vi "QPlus_Analyzer 2.0.vi"() -> ()   [LabVIEW 2016]
uses:
  <instrlib>/Stanford Research 830/Public/Data/Read (1 Parameter).vi
  <vilib>/express/express shared/transition.llb/Dynamic To Waveform Array.vi
  <vilib>/express/express signal manip/GetorSetDDTAttributes/Set DDT Attributes/SetT0.vi
  <vilib>/express/express shared/transition.llb/Waveform Array To Dynamic.vi
  <vilib>/express/express signal manip/GetorSetDDTAttributes/Set DDT Attributes/Set DDT Properties.xnode
  <instrlib>/Stanford Research 830/Stanford Research 830.lvlib
  <instrlib>/Agilent 3352X Series/Agilent 3352X Series.lvlib
panel:
  out "Y Signal":cluster{"Y":dbl[], "Y":dbl[]}[](graph)
  out "X Signal":cluster{"Y":dbl[], "Y":dbl[]}[](graph)
  in  "Reference name":refnum<visa-resource-name>
  in  "VISA resource name":refnum<visa-resource-name>
  in  "Sensitivity (26: 1 V/uA)":i8(ring)=26 items=["Auto Gain"=-1, "2 nV/fA"=0, "5 nV/fA"=1, "10 nV/fA"=2, "20 nV/fA"=3, "50 nV/fA"=4, "100 nV/fA"=5, "200 nV/fA"=6, "500 nV/fA"=7, "1 uV/pA"=8, "2 uV/pA"=9, "5 uV/pA"=10, "10 uV/pA"=11, "20 uV/pA"=12, "50 uV/pA"=13, "100 uV/pA"=14, "200 uV/pA"=15, "500 uV/pA"=16, "1 mV/nA"=17, "2 mV/nA"=18, "5 mV/nA"=19, "10 mV/nA"=20, "20 mV/nA"=21, "50 mV/nA"=22, "100 mV/nA"=23, "200 mV/nA"=24, "500 mV/mA"=25, "1 V/uA"=26]
  in  "Time Constant (8: 100ms)":u16(ring)=8 items=["10 us", "30 us", "100 us", "300 us", "1 ms", "3 ms", "10 ms", "30 ms", "100 ms", "300 ms", "1 s", "3 s", "10 s", "30 s", "100 s", "300 s", "1 ks", "3 ks", "10 ks", "30 ks"]
  in  "Save File Name":path=path "G:/UCB/Instruments/tip making/Qplus AFM tip making/qplus test/Caihong/CJ39.xlsx" caption="Filename"
  in  "Time Between Points (sec)":dbl=0.05 format="%#_1f"
  in  "Sine Output Amplitude (1 V)":dbl=1.0
  in  "Starting Frequency (Hz)":dbl=32000.0
  in  "Final Frequency (Hz)":dbl=33000.0
  in  "Step Size (Hz)":dbl=10.0
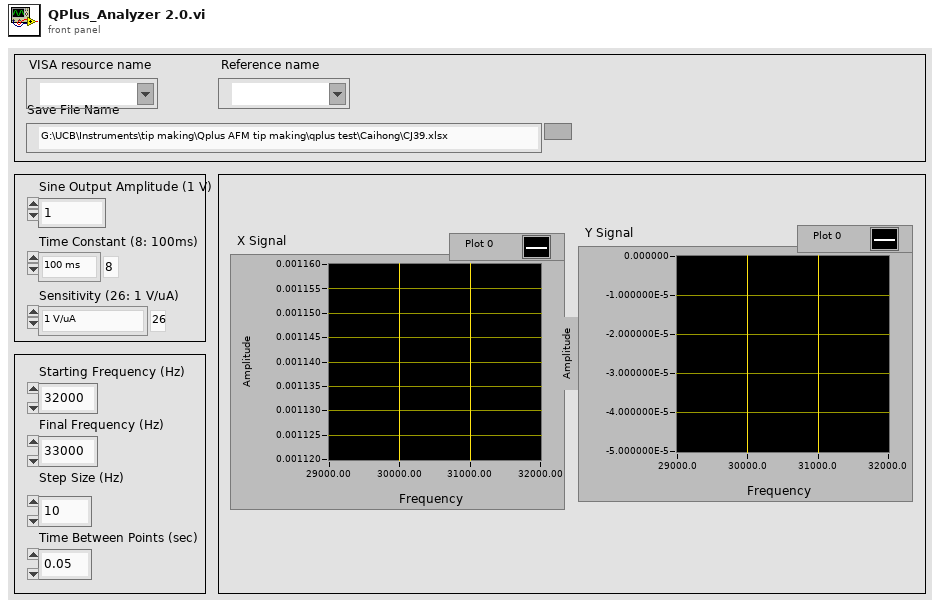
[diagram p1: front panel]
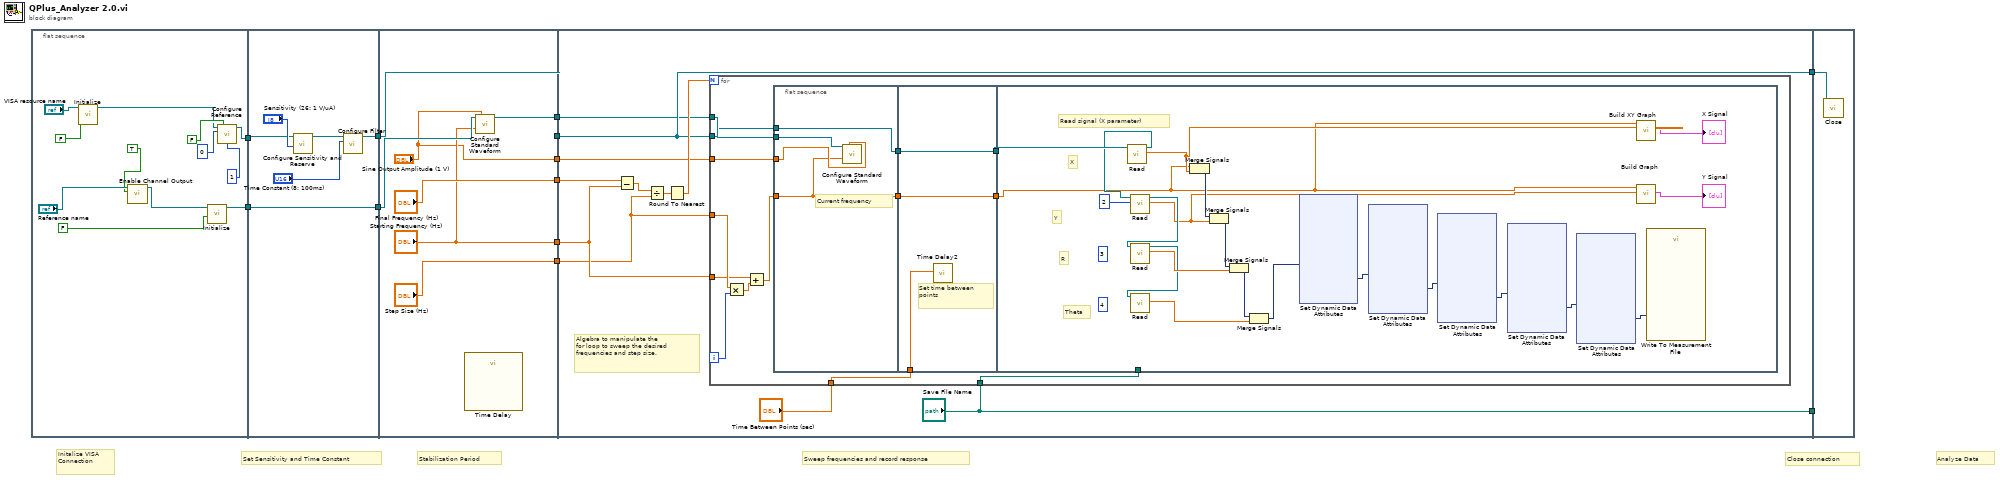
[diagram p0: block diagram]
diagram:
  # "Stabilization Period"
  # "Analyze Data"
  # "Close connection"
  # "Sweep frequencies and record response"
  # "Set Sensitivity and Time Constant"
  # "Initalize VISA\nConnection"
  n1 = flat-sequence {
    tunnel: [w20] -> w12
    tunnel: [w21] -> w2
    tunnel: [w27] -> w9
    tunnel: w12 -> [w26]
    tunnel: [w25] -> w3
    tunnel: w2 -> [w25]
    tunnel: w9 -> [w35]
    tunnel: [w35] -> w8
    tunnel: ["Starting Frequency (Hz)"] -> w7
    tunnel: ["Final Frequency (Hz)"] -> w6
    tunnel: ["Step Size (Hz)"] -> w5
    tunnel: ["Sine Output Amplitude (1 V)"] -> w4
    tunnel: w3 -> [w33]
    tunnel: [w34] -> w1
    tunnel: w8 -> [w45]
    tunnel: [w45] -> w11
    tunnel: ["Save File Name"] -> w10
    tunnel: w7 -> [w42]
    tunnel: w6 -> [w41]
    tunnel: w5 -> [w40]
    tunnel: w4 -> [w39]
    tunnel: w1 -> [w38]
    tunnel: w11 -> [w161]
    tunnel: w10 -> [_]
    frame #0 {
      n2 = call <instrlib>:"Initialize.vi"("Reset (True)"=FALSE, "VISA resource name"="VISA resource name") -> ("VISA resource name out"=w13:refnum<visa-resource-name>)  [unwired: 8 in, 1 out]
      n3 = call <instrlib>:"Enable Channel Output.vi"("Enable Output (T: Enable)"=TRUE, "VISA resource name"="Reference name") -> ("VISA resource name out"=w15:refnum<visa-resource-name>)  [unwired: 8 in, 1 out]
      n4 = call <instrlib>:"Initialize.vi"("Reset (Enable)"=FALSE, "VISA resource name"=w15) -> ("VISA resource name out"=w21:refnum<visa-resource-name>)  [unwired: 8 in, 1 out]
      n5 = call "Configure Reference.vi"("VISA resource name"=w13, "Auto Phase (T: Enabled)"=FALSE, "Reference Source (1: Internal)"=0, "External Reference Trigger (0: Sine Zero Crossing)"=1) -> ("VISA resource name out"=w20:refnum<visa-resource-name>)  [unwired: 10 in, 1 out]
    }
    frame #1 {
      n6 = call <instrlib>:"Configure Sensitivity and Reserve.vi"("Sensitivity (-1: Auto gain)"="Sensitivity (26: 1 V/uA)", "VISA resource name"=w26) -> ("VISA resource name out"=w29:refnum<visa-resource-name>)  [unwired: 8 in, 1 out]
      n7 = call <instrlib>:"Configure Filter.vi"("Time Constant (8: 100ms)"="Time Constant (8: 100ms)", "VISA resource name"=w29) -> ("VISA resource name out"=w27:refnum<visa-resource-name>)  [unwired: 8 in, 1 out]
    }
    frame #2 {
      n8 = call "Time Delay"() -> ()  [unwired: 11 in, 1 out]
      n9 = call <instrlib>:"Configure Standard Waveform.vi"("VISA resource name"=w33, "Amplitude (0.1 Vpp)"="Sine Output Amplitude (1 V)", "Frequency/Sample Rate/Bandwidth (1000 Hz)"="Starting Frequency (Hz)") -> ("VISA resource name out"=w34:refnum<visa-resource-name>)  [unwired: 11 in, 1 out]
    }
    frame #3 {
      # "Algebra to manipulate the\nfor loop to sweep the desired\nfrequencies and step size."
      n10 = Subtract(x=w41, y=w42) -> (x-y=w48:dbl)
      n11 = Divide(x=w48, y=w40) -> (x/y=w47:dbl)
      n12 = Round To Nearest(number=w47) -> (nearest integer value=w46:dbl)
      n13 = for {
        N: w46 -> [_]
        tunnel: w40 -> [w61]
        tunnel: w42 -> [w59]
        tunnel: w45 -> [w50]
        tunnel: "Time Between Points (sec)" -> [w52]
        tunnel: "Save File Name" -> [w57]
        tunnel: w39 -> [w56]
        tunnel: w38 -> [w51]
        i -> [w62]
        n14 = Multiply(x=w61, y=w62) -> (x*y=w60:dbl)
        n15 = Add(x=w59, y=w60) -> (x+y=w58:dbl)
        n16 = flat-sequence {
          tunnel: [w63] -> w54
          tunnel: w58 -> [w63]
          tunnel: w56 -> [w65]
          tunnel: w51 -> [w64]
          tunnel: w50 -> [w66]
          tunnel: [w66] -> w49
          tunnel: [w69] -> w55
          tunnel: w54 -> [w68]
          tunnel: [w68] -> w53
          tunnel: w52 -> [w67]
          tunnel: w49 -> [w69]
          tunnel: w55 -> [w90]
          tunnel: w53 -> [w77]
          tunnel: w57 -> [_]
          frame #0 {
            # "Current frequency"
            n17 = call <instrlib>:"Configure Standard Waveform.vi"("VISA resource name"=w64, "Amplitude (0.1 Vpp)"=w65, "Frequency/Sample Rate/Bandwidth (1000 Hz)"=w63) -> ()  [unwired: 11 in, 2 out]
          }
          frame #1 {
            # "Set time between\npoints"
            n18 = call "Time Delay2"("Delay Time (s)"=w67) -> ()  [unwired: 10 in, 1 out]
          }
          frame #2 {
            (unwired) 4
            (unwired) 3
            # "X"
            # "Y"
            # "R"
            # "Theta"
            # "Read signal (X parameter)"
            n19 = call-poly <instrlib>:"Read.vi"("VISA resource name"=w90) -> ("Measurement"=w80:dbl, "VISA resource name out"=w83:refnum<visa-resource-name>)  [unwired: 8 in, 1 out]
            n20 = call-poly <instrlib>:"Read.vi"("Parameter (1: X)"=2, "VISA resource name"=w83) -> ("Measurement"=w76:dbl, "VISA resource name out"=w82:refnum<visa-resource-name>)  [unwired: 7 in, 1 out]
            n21 = call-poly <instrlib>:"Read.vi"("VISA resource name"=w82) -> ("Measurement"=w86:dbl, "VISA resource name out"=w81:refnum<visa-resource-name>)  [unwired: 8 in, 1 out]
            n22 = call-poly <instrlib>:"Read.vi"("VISA resource name"=w81) -> ("Measurement"=w84:dbl)  [unwired: 8 in, 2 out]
            n23 = Merge Signals(w77, w80) -> (w88:dynamicdata)
            n24 = Merge Signals(w88, w76) -> (w87:dynamicdata)
            n25 = Merge Signals(w87, w86) -> (w85:dynamicdata)
            n26 = Merge Signals(w85, w84) -> (w75:dynamicdata)
            n27 = xnode "Set Dynamic Data Attributes"("Signals In"=w75) -> ("Signals Out"=w74:dynamicdata)  [unwired: 3 in, 1 out]
            n28 = xnode "Set Dynamic Data Attributes"("Signals In"=w74) -> ("Signals Out"=w73:dynamicdata)  [unwired: 3 in, 1 out]
            n29 = xnode "Set Dynamic Data Attributes"("Signals In"=w73) -> ("Signals Out"=w72:dynamicdata)  [unwired: 3 in, 1 out]
            n30 = xnode "Set Dynamic Data Attributes"("Signals In"=w72) -> ("Signals Out"=w71:dynamicdata)  [unwired: 3 in, 1 out]
            n31 = xnode "Set Dynamic Data Attributes"("Signals In"=w71) -> ("Signals Out"=w70:dynamicdata)  [unwired: 3 in, 1 out]
            n32 = call "Build XY Graph"("Y Input"=w80, "X Input"=w77) -> ("XY Graph"=→"X Signal":cluster{"Y":dbl[], "Y":dbl[]}[])  [unwired: 3 in, 6 out]
            n33 = call "Build Graph"("Y Input"=w76, "X Input"=w77) -> ("XY Graph"=→"Y Signal":cluster{"Y":dbl[], "Y":dbl[]}[])  [unwired: 3 in, 6 out]
            n34 = call "Write To Measurement File"("Signals"=w70) -> ()  [unwired: 16 in, 3 out]
          }
        }
      }
    }
    frame #4 {
      n35 = call <instrlib>:"Close.vi"("VISA resource name"=w161) -> ()  [unwired: 10 in, 1 out]
    }
  }
